vi "Stop.vi"(0 "reference in":refnum<class "J1939-22_Engine.lvclass">, 5 "Error In":errorcluster) -> (14 "reference out":refnum<class "J1939-22_Engine.lvclass">, 19 "Error Out":errorcluster)   [LabVIEW 2021, in "J1939-22_Engine.lvclass"]
uses:
  J1939-22_Engine.lvclass
  <vilib>/xnet/xnet.llb/XNET Database Close (Database).vi
  J1939-22_Database_class/J1939-22_Database.lvclass
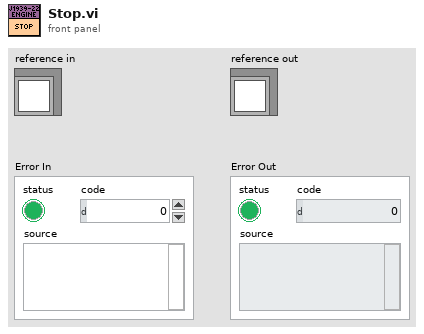
[diagram p1: front panel]
types:
  T1 = typedef "J1939-22_Engine.lvclass/ObjectAttributes.ctl" = cluster{"Data":T2[], "DTCs":T15[], "XNET.Settings.Database":refnum<k21>, "J1939-22_Database":refnum<class "J1939-22_Database.lvclass">}
  T2 = typedef "J1939 Addon Engine.lvlib/Protocol.XNET Refs.ctl" = cluster{"Network":T3, "Incoming.Use":bool, "Incoming.Session":refnum<k21>, "Incoming.Refs":T4[], "Incoming.Values":dbl[], "Outgoing.Frames":T6[], "Outgoing.Initialize":bool, "Outgoing.Refs":T4[], "Outgoing.Values":dbl[], "Request.Table":refnum<k33>, "Timing.Use":bool, "Timing.Index":i32[], "Timing.Refs":T4[], "Timing.Values":dbl[], "Disable.Refs":T4[], "Disable.Values":dbl[], "Trigger.Refs":T4[], "Trigger.Values":dbl[], "Outgoing.Frames.CountersAndProtections":T8[]}
  T3 = typedef "J1939 Addon Shared.lvlib/Monitor Settings.ctl" = cluster{"Address":u8, "Name":u64, "Include DA":bool, "Force SA":bool}
  T4 = typedef "Custom Device API.lvlib/Block Data Reference.ctl" = cluster{"Data Reference":T5, "Offset":u64, "Length":u64}
  T5 = typedef "Custom Device API.lvlib/Data Reference.ctl" = i32
  T6 = typedef "J1939 Addon Engine.lvlib/Main.Outgoing.Frame.Settings.ctl" = cluster{"Offset":u32, "Length":u32, "Cyclic":bool, "Disable.Index":i32, "Disable":bool, "Trigger":T7, "Trigger.Index":i32, "Session":refnum<k21>}
  T7 = typedef "J1939 Addon Shared.lvlib/Outgoing Event Trigger Types.ctl" = enum16{"Channel value change", "Trigger channel (not zero)", "Channel value change or trigger channel (not zero)", "Trigger channel (any value change)", "Channel value change or trigger channel (any value change)"}
  T8 = typedef "Protection and Counter Support Shared.lvlib/Exported Frame Settings.ctl" = cluster{"Type":T9, "Frame ID":u32, "Payload Length":u32, "Signal XNET Paths":string[], "Frame.PrevData":dbl[], "VS Offset":i32, "VS Length":i32, "Generation Period":u32, "Has Protection?":bool, "Protection Configurations":T10[], "Has Counter":bool, "Counter Configurations":T13[], "Has Disable?":bool, "Disable VS Index":i32, "Transmit Trigger":T14, "Trigger VS Index":i32}
  T9 = typedef "Protection and Counter Support Shared.lvlib/Exported Frame Type.ctl" = enum16{"Periodic", "Event", "Periodic/Event"}
  T10 = typedef "Protection and Counter Support Shared.lvlib/Exported Protection Settings.ctl" = cluster{"Protection Frame Index":i32, "Protection Type":T11, "Data Indeces":i32[], "Initialized Data Array":dbl[], "Protection Signal XNET Paths":string[], "CRC Channels":T12[], "Protection VS Update Index":i32, "Override Index":i32, "Override Value Index":i32}
  T11 = typedef "Protection and Counter Support Shared.lvlib/Protection Type.ctl" = enum16{"Arb ID + Bytes Checksum with Inversion", "Arb ID + Bytes CRC with Inversion", "Reversed Raw Signal Checksum with Inversion", "Concatenated Two's Compliment"}
  T12 = typedef "Protection and Counter Support Shared.lvlib/XNET Signal Configuration.ctl" = cluster{"Start Bit":i32, "Name":string, "Number of bits":i32, "Scale":dbl, "Offset":dbl, "Data Type":u32, "Counter":bool}
  T13 = typedef "Protection and Counter Support Shared.lvlib/Exported Counter Settings.ctl" = cluster{"Frame Index":i32, "Max Count":dbl, "VS Index":i32, "Bit Length":i64, "Override Index":i32, "Override Value Index":i32}
  T14 = typedef "Protection and Counter Support Shared.lvlib/Exported Event Trigger Type.ctl" = enum16{"Channel value change", "Trigger channel (not zero)", "Channel value change or trigger channel (not zero)", "Trigger channel (any value change)", "Channel value change or trigger channel (any value change)"}
  T15 = typedef "J1939 Addon Engine.lvlib/Engine.DTC Settings.ctl" = cluster{"Data":T16, "FIFOs":T17}
  T16 = typedef "J1939 Addon Shared.lvlib/Compiled Simulated Settings.ctl" = cluster{"DM1.Ref":T4[], "DM1.Value":dbl[], "DM1.Enable.Ref":T4[], "DM1.Enable.Value":dbl[], "DM2.Ref":T4[], "DM2.Value":dbl[], "DM2.Enable.Ref":T4[], "DM2.Enable.Value":dbl[]}
  T17 = typedef "J1939 Addon Engine.lvlib/Engine.DTC FIFOs.ctl" = cluster{"DM1.Data":refnum<k33>, "DM1.Enable":refnum<k33>, "DM2.Data":refnum<k33>, "DM2.Enable":refnum<k33>, "DM1.Reset":refnum<k33>, "DM2.Reset":refnum<k33>}
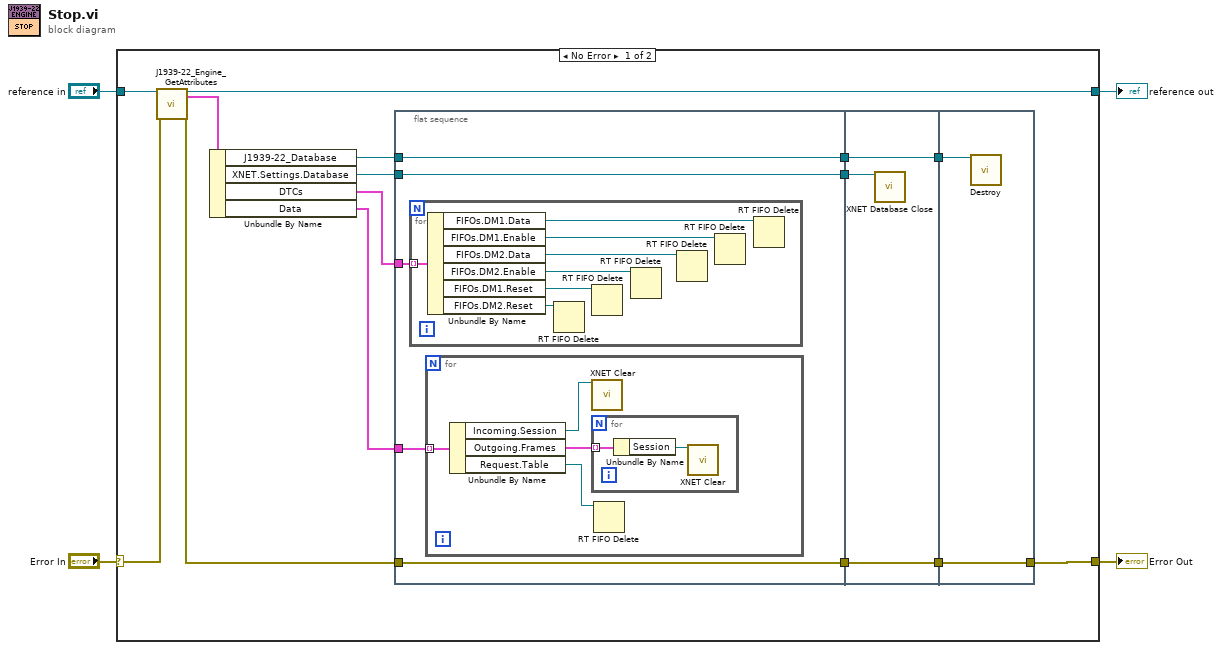
[diagram p0: block diagram]
diagram:
  n1 = case shown="No Error" "Error In" {
    selector: "Error In" -> [w19 w44]
    tunnel: [w5 w44] -> w3
    tunnel: [w17 w43] -> w1
    tunnel: "reference in" -> [w18 w43]
    frame No Error {
      n2 = call "J1939-22_Engine_GetAttributes.vi"("reference in"=w18, "Error In"=w19) -> ("reference out"=w17:refnum<class "J1939-22_Engine.lvclass">, "Data"=w13:T1, "Error Out"=w10:errorcluster)  [unwired: 14 in, 1 out]
      n3 = Unbundle By Name(w13) -> ("J1939-22_Database"=w9:refnum<class "J1939-22_Database.lvclass">, "XNET.Settings.Database"=w12:refnum<k21>, "DTCs"=w11:T15[], "Data"=w6:T2[])
      n4 = flat-sequence {
        tunnel: w10 -> [w24]
        tunnel: w12 -> [w22]
        tunnel: [w24] -> w16
        tunnel: [w22] -> w15
        tunnel: w11 -> [w23]
        tunnel: w9 -> [w21]
        tunnel: [w21] -> w7
        tunnel: w6 -> [w20]
        tunnel: w16 -> [w40]
        tunnel: w15 -> [w39]
        tunnel: [w40] -> w14
        tunnel: [w38] -> w8
        tunnel: w7 -> [w38]
        tunnel: [w42] -> w5
        tunnel: w14 -> [w42]
        tunnel: w8 -> [w41]
        frame #0 {
          n5 = for {
            tunnel: w23 -> [w31] mode=indexing
            n6 = Unbundle By Name(w31) -> ("FIFOs.DM1.Data"=w30:refnum<k33>, "FIFOs.DM1.Enable"=w29:refnum<k33>, "FIFOs.DM2.Data"=w28:refnum<k33>, "FIFOs.DM2.Enable"=w25:refnum<k33>, "FIFOs.DM1.Reset"=w26:refnum<k33>, "FIFOs.DM2.Reset"=w27:refnum<k33>)
            n7 = RT FIFO Delete(0:w27) -> ()  [unwired: 2 in, 1 out]
            n8 = RT FIFO Delete(0:w26) -> ()  [unwired: 2 in, 1 out]
            n9 = RT FIFO Delete(0:w25) -> ()  [unwired: 2 in, 1 out]
            n10 = RT FIFO Delete(0:w28) -> ()  [unwired: 2 in, 1 out]
            n11 = RT FIFO Delete(0:w29) -> ()  [unwired: 2 in, 1 out]
            n12 = RT FIFO Delete(0:w30) -> ()  [unwired: 2 in, 1 out]
          }
          n13 = for {
            tunnel: w20 -> [w33] mode=indexing
            n14 = Unbundle By Name(w33) -> ("Incoming.Session"=w35:refnum<k21>, "Outgoing.Frames"=w34:T6[], "Request.Table"=w32:refnum<k33>)
            n15 = call <vilib>:"XNET Clear.vi"("session in"=w35) -> ()  [unwired: 14 in, 1 out]
            n16 = for {
              tunnel: w34 -> [w37] mode=indexing
              n17 = Unbundle By Name(w37) -> ("Session"=w36:refnum<k21>)
              n18 = call <vilib>:"XNET Clear.vi"("session in"=w36) -> ()  [unwired: 14 in, 1 out]
            }
            n19 = RT FIFO Delete(0:w32) -> ()  [unwired: 2 in, 1 out]
          }
        }
        frame #1 {
          n20 = call-poly <vilib>:"XNET Database Close.vi"("database in"=w39) -> ()  [unwired: 14 in, 1 out]
        }
        frame #2 {
          n21 = call-dynamic "Destroy.vi"("reference in"=w41) -> ()  [unwired: 17 in, 2 out]
        }
      }
    }
    frame Error {
    }
  }
  "Error Out" <- w3
  "reference out" <- w1
